vi "uEye_Control_V1.vi"() -> ()   [LabVIEW 2014]
uses:
  Focus Lock/Controls/Standard Action for Camera Control.ctl
  Focus Lock/Controls/Standard Action for Focus Lock.ctl
  C:/Program Files (x86)/National Instruments/LabVIEW 2014/instr.lib/IDS/ueye.NET/uEyeDotNet.dll
  Program Files (x86)/National Instruments/LabVIEW 2014/instr.lib/IDS/ueye.NET/uEyeDotNet.dll
panel:
  in  "Exit":bool
  in  "Exposure Time (ms)":dbl(slide) scale=0.06..1.0
  out "Camera Image":u8[][](graph)
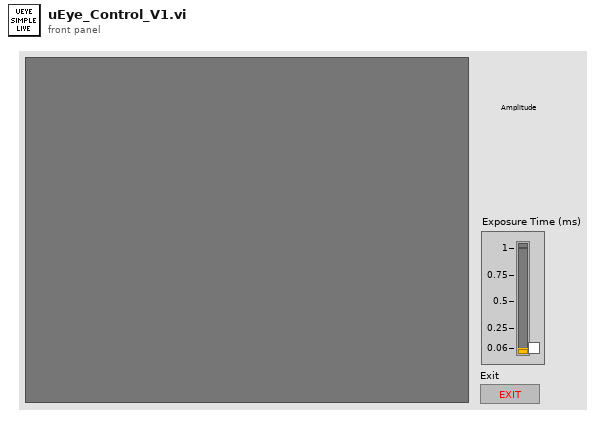
[diagram p1: front panel]
types:
  T1 = typedef "Standard Action for Camera Control.ctl" = enum16{"Read", "Setting", "Switch", "Initialization", "Exit"}
  T2 = typedef "Standard Action for Focus Lock.ctl" = enum16{"Read", "Write"}
  T3 = typedef "Camera Control.ctl" = cluster{"Pixel Clock (MHz)":i32, "Exposure Time (ms)":dbl, "Frame Rate (fps)":dbl, "ROI Half Width":i32, "Switch":bool}
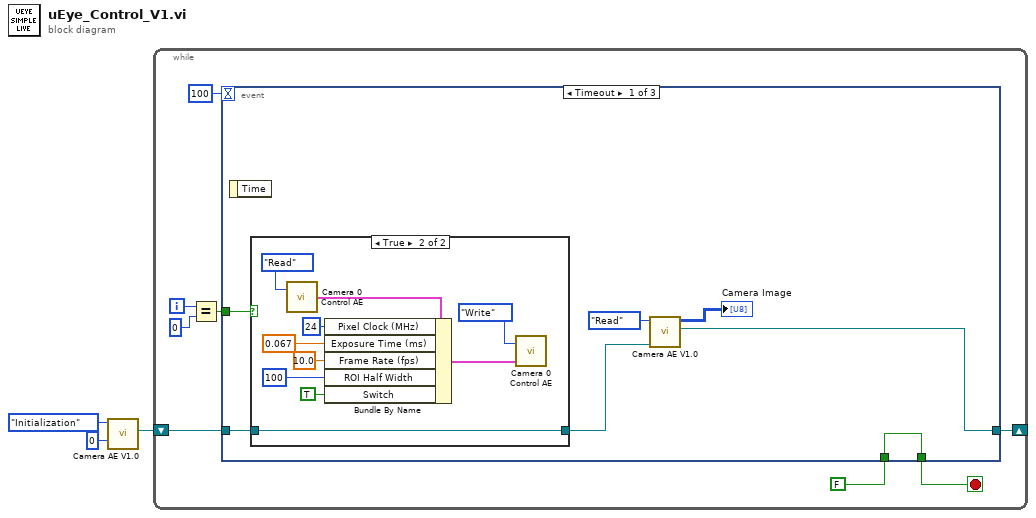
[diagram p0: block diagram]
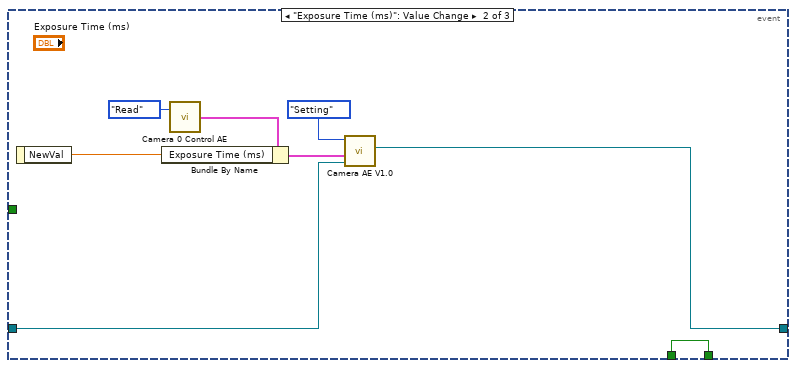
[diagram p3: hidden frame]
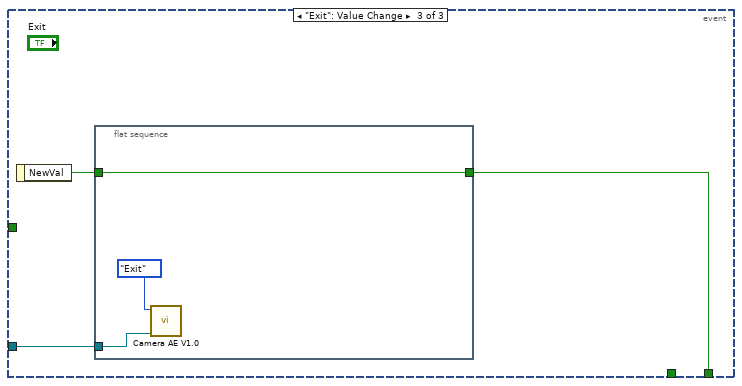
[diagram p4: hidden frame]
diagram:
  n1 = call "Camera AE V1.0.vi"("Camera ID"=0, "Action"=Standard_Action_for_Camera_Control."Initialization") -> ("Reference Out"=w1:refnum<k24>)  [unwired: 4 in, 3 out]
  n2 = while {
    shift-right: [w8] -> _
    shift-left: w1 -> [w9]
    i -> [w7]
    stop <- w10 stop-if-true
    n3 = Equal?(x=w7, y=0) -> (x = y?=w5:bool)
    n4 = event shown="[0] Timeout" {
      selector: _ -> [_ _ _]
      dyn-events: _ -> [_ _ _]
      timeout: 100 -> [_ _ _]
      tunnel: FALSE -> [w18 w30 _]
      tunnel: [w18 w30 w38] -> w10
      tunnel: w9 -> [w14 w32 w40]
      tunnel: [w17 w31 _] -> w8
      tunnel: w5 -> [w15 _ _]
      event Timeout {
        n5 = event-data() -> ()  [unwired: 1 in, 1 out]
        n6 = case shown="True" w15 {
          tunnel: [w19 w29] -> w13
          tunnel: w14 -> [w19 w29]
          frame False {
          }
          frame True {
            n7 = call "Camera 0 Control AE.vi"("Action"=Standard_Action_for_Focus_Lock."Read") -> ("Camera Control Output"=w27:T3)  [unwired: 1 in]
            n8 = Bundle By Name(cluster=w27, "Pixel Clock (MHz)"=24, "Exposure Time (ms)"=0.067, "Frame Rate (fps)"=10.0, "ROI Half Width"=100, "Switch"=TRUE) -> (w21:T3)
            n9 = call "Camera 0 Control AE.vi"("Camera Control Input"=w21, "Action"=Standard_Action_for_Focus_Lock."Write") -> ()  [unwired: 1 out]
          }
        }
        n10 = call "Camera AE V1.0.vi"(".NET (Reference)"=w13, "Action"=Standard_Action_for_Camera_Control."Read") -> ("Reference Out"=w17:refnum<k24>, "Array"=→"Camera Image":u8[][])  [unwired: 4 in, 2 out]
      }
      event "Exposure Time (ms)": Value Change {
        n11 = event-data() -> ("NewVal"=w35:dbl)  [unwired: 1 in]
        n12 = call "Camera 0 Control AE.vi"("Action"=Standard_Action_for_Focus_Lock."Read") -> ("Camera Control Output"=w36:T3)  [unwired: 1 in]
        n13 = Bundle By Name(cluster=w36, "Exposure Time (ms)"=w35) -> (w34:T3)
        n14 = call "Camera AE V1.0.vi"(".NET (Reference)"=w32, "Camera Control In"=w34, "Action"=Standard_Action_for_Camera_Control."Setting") -> ("Reference Out"=w31:refnum<k24>)  [unwired: 3 in, 3 out]
      }
      event "Exit": Value Change {
        n15 = event-data() -> ("NewVal"=w39:bool)  [unwired: 1 in]
        n16 = flat-sequence {
          tunnel: w40 -> [w43]
          tunnel: [w41] -> w38
          tunnel: w39 -> [w41]
          frame #0 {
            n17 = call "Camera AE V1.0.vi"(".NET (Reference)"=w43, "Action"=Standard_Action_for_Camera_Control."Exit") -> ()  [unwired: 4 in, 4 out]
          }
        }
      }
    }
  }
